vi "Write Session.TCPIP.KeepAliveTimeout.vi"(8 "error in (no error)":errorcluster, 10 "Session.TCPIP.KeepAliveTimeout":dbl, 11 "SLSC Local in":refnum<class "SLSC Local.lvclass">) -> (0 "error out":errorcluster, 3 "SLSC Local out":refnum<class "SLSC Local.lvclass">)   [LabVIEW 2015, in "SLSC Local.lvclass"]
uses:
  SLSC Local.lvclass
  <resource>/objmgr/slsc.rc
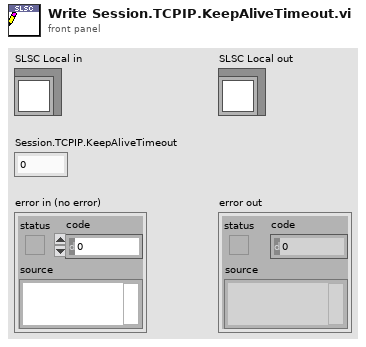
[diagram p1: front panel]
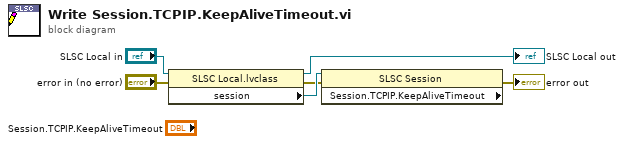
[diagram p0: block diagram]
diagram:
  n1 = property class="SLSC Local.lvclass"(reference="SLSC Local in", error in="error in (no error)") -> (reference out=→"SLSC Local out":refnum<class "SLSC Local.lvclass">, error out=w5:errorcluster, "session"=w6:refnum<k21>)
  n2 = property class="SLSC Session" props=["Session.TCPIP.KeepAliveTimeout"](reference=w6, error in=w5) -> (error out=→"error out":errorcluster)  [unwired: 2 out]
